vi "Reset.vi"(7 "Reconnect \nwait time [ms]":u32=2000, 8 "Error In":errorcluster, 10 "Reset Target":T7, 11 "LINX Resource":T1) -> (0 "Error Out":errorcluster, 3 "LINX Resource out":T1)   [LabVIEW 2019, in "LINXx.lvlib"]
doc: "Reset the device or one of its peripherals.\nFor whole board reset, VI attempts to reestablish communication after the reset."
uses:
  LINXx.lvlib
  Public/Reset Target.ctl
  <vilib>/MakerHub/LINX/Private/Type Defs/LINX Ref.ctl
  <vilib>/MakerHub/LINX/Private/Type Defs/Platform.ctl
  <vilib>/MakerHub/LINX/Private/Type Defs/Interface.ctl
  <vilib>/MakerHub/LINX/Private/Device/Type Defs/LINX Device Config.ctl
  <vilib>/MakerHub/LINX/Private/Device/Type Defs/TCP Config.ctl
  <vilib>/MakerHub/LINX/Private/Device/Type Defs/Channels.ctl
  <vilib>/MakerHub/LINX/Private/Type Defs/User Platform.ctl
  <vilib>/MakerHub/LINX/Public/Initialize.vi
  <vilib>/MakerHub/LINX/LMH-LINX.lvlib
  <vilib>/MakerHub/LINX/Private/Device/Device.lvlib
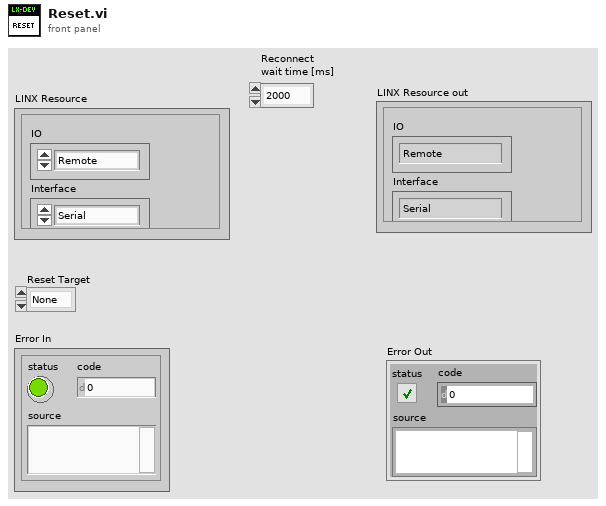
[diagram p1: front panel]
types:
  T1 = typedef "LMH-LINX.lvlib/LINX Ref.ctl" = cluster{"IO":T2, "Interface":T3, "LINX Device Config":T4}
  T2 = typedef "LMH-LINX.lvlib/Platform.ctl" = enum16{"Remote", "Local"}
  T3 = typedef "LMH-LINX.lvlib/Interface.ctl" = enum16{"Serial", "TCP"}
  T4 = typedef "LMH-LINX.lvlib/Device.lvlib/LINX Device Config.ctl" = cluster{"Interface":T3, "COM Port":refnum<visa-resource-name>, "TCP Configuration":T5, "Device Family":u8, "Device ID":u8, "Device Name":string, "TCP Ref":refnum<k5>, "Channels":T6}
  T5 = typedef "LMH-LINX.lvlib/Device.lvlib/TCP Config.ctl" = cluster{"IP Address":string, "Port":u16}
  T6 = typedef "LMH-LINX.lvlib/Channels.ctl" = cluster{"DI":u8[], "DO":u8[], "AI":u8[], "AO":u8[], "PWM":u8[], "QE":u8[], "UART":u8[], "I2C 2":u8[], "SPI":u8[], "CAN":u8[], "Servo":u8[], "AI Ref (V)":dbl, "AI Resolution (Bits)":u8, "AO Ref (V)":dbl, "AO Resolution (Bits)":u8}
  T7 = typedef "LINXx.lvlib/Reset Target.ctl" = enum16{"None", "Serial", "TCP", "Board"}
  T8 = typedef "LMH-LINX.lvlib/User Platform.ctl" = enum16{"Default", "Remote", "Local"}
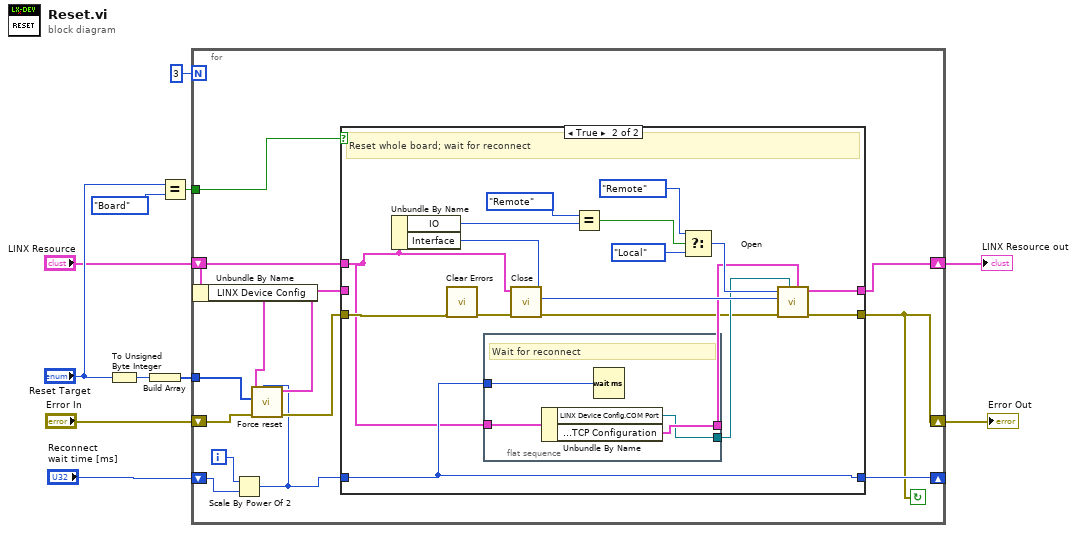
[diagram p0: block diagram]
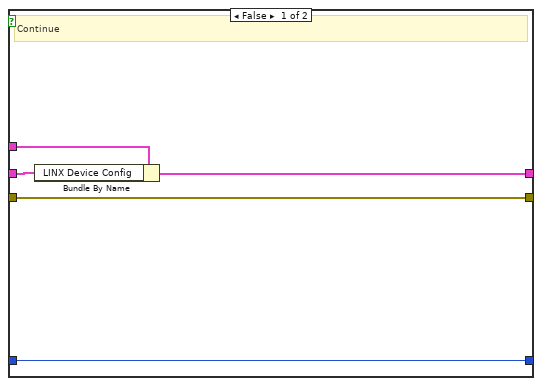
[diagram p2: hidden frame]
diagram:
  n1 = To Unsigned Byte Integer(number="Reset Target") -> (unsigned 8bit integer=w11:u8)
  n2 = Build Array(w11) -> (w10:u8[])
  n3 = Equal?(x="Reset Target", y=Reset_Target."Board" ("Reset Target 2")) -> (x = y?=w6:bool)
  n4 = for {
    N: 3 -> [_]
    tunnel: w10 -> [w24]
    tunnel: w6 -> [w21]
    shift-right: [w14] -> w5
    shift-left: "Error In" -> [w23]
    shift-right: [w20] -> w4
    shift-left: "LINX Resource" -> [w18]
    shift-right: [w15] -> _
    shift-left: "Reconnect \nwait time [ms]" -> [w12]
    i -> [w13]
    stop <- w14 continue-if-true
    n5 = Unbundle By Name(w18) -> ("LINX Device Config"=w17:T4)
    n6 = Scale By Power Of 2(n=w13, x=w12) -> (x*2^n=w16:u32)
    n7 = call "Force reset.vi"("Timeout (100 ms)"=w16, "Error In"=w23, "Reset Target"=w24, "LINX Device Config"=w17) -> ("Error Out"=w22:errorcluster, "Dup LINX Device Config"=w19:T4)  [unwired: 6 in]
    n8 = case shown="True" w21 {
      tunnel: w22 -> [w29 w33]
      tunnel: [w29 w45] -> w14
      tunnel: [w27 w44] -> w20
      tunnel: w19 -> [w26 _]
      tunnel: w18 -> [w28 w31]
      tunnel: w16 -> [w25 w34]
      tunnel: [w25 w34] -> w15
      frame False {
        # "Continue"
        n9 = Bundle By Name(cluster=w28, "LINX Device Config"=w26) -> (w27:T1)
      }
      frame True {
        # "Reset whole board; wait for reconnect"
        n10 = Unbundle By Name(w31) -> ("IO"=w38:T2, "Interface"=w37:T3)
        n11 = call <vilib>:"Clear Errors.vi"("error in (no error)"=w33) -> ("error out"=w32:errorcluster)  [unwired: 5 in, 1 out]
        n12 = flat-sequence {
          tunnel: [w49] -> w36
          tunnel: [w48] -> w35
          tunnel: w31 -> [w47]
          tunnel: w34 -> [w46]
          frame #0 {
            # "Wait for reconnect"
            n13 = Unbundle By Name(w47) -> ("LINX Device Config.COM Port"=w48:refnum<visa-resource-name>, "LINX Device Config.TCP Configuration"=w49:T5)
            n14 = Wait (ms)(milliseconds to wait=w46) -> ()  [unwired: 1 out]
          }
        }
        n15 = call <vilib>:"Close.vi"("Error In"=w32, "LINX Resource"=w31) -> ("Error Out"=w30:errorcluster)  [unwired: 9 in]
        n16 = Equal?(x=Platform."Remote" ("IO"), y=w38) -> (x = y?=w43:bool)
        n17 = Select(t=User_Platform."Remote" ("IO"), s=w43, f=User_Platform."Local") -> (s? t:f=w39:T8)
        n18 = call-poly <vilib>:"Open.vi"("TCP Configuration"=w36, "Serial Port"=w35, "Error In"=w30, "Interface"=w37, "IO"=w39) -> ("Error Out"=w45:errorcluster, "LINX Resource"=w44:T1)  [unwired: 4 in, 1 out]
      }
    }
  }
  "LINX Resource out" <- w4
  "Error Out" <- w5
